vi "Tree Strings.vi"(8 "error in (no error)":errorcluster, 11 "Folder Item in":refnum<class "Folder Item.lvclass">) -> (0 "error out":errorcluster, 1 "Child Text":string[](array[string]), 2 "Left Cell String":string, 3 "Folder Item out":refnum<class "Folder Item.lvclass">, 5 "Child Tag":string)   [LabVIEW 2020, in "BetterDragAndDropDemo.lvlib" / "Folder Item.lvclass"]
uses:
  Folder Item.lvclass
  Folder Item.lvclass/Folder Item.ctl
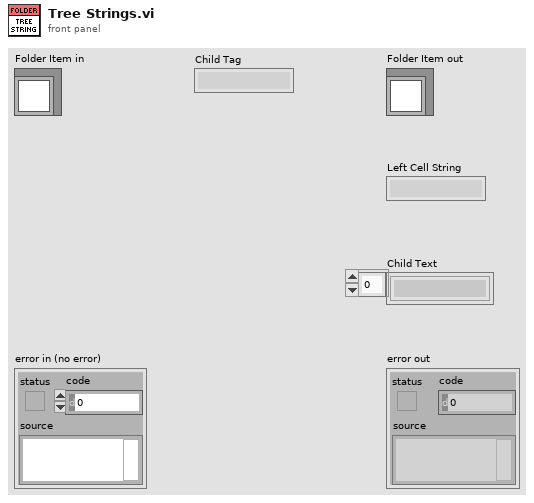
[diagram p1: front panel]
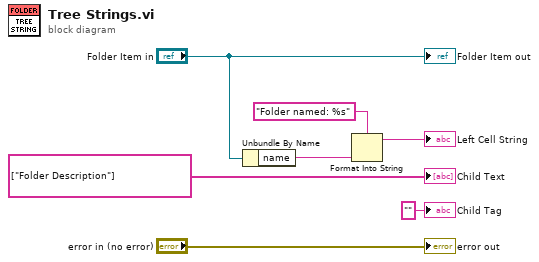
[diagram p0: block diagram]
diagram:
  n1 = Unbundle By Name("Folder Item in") -> ("name"=w2:string)
  n2 = Format Into String(format string="Folder named: %s", w2) -> (resulting string=→"Left Cell String":string)  [unwired: 2 in, 1 out]
  "error out" <- "error in (no error)"
  "Folder Item out" <- "Folder Item in"
  "Child Text" <- string[] ["Folder Description"] ("Child Text")
  "Child Tag" <- "" ("Child Tag")
